vi "svx_Waterfall ZUnitsToIndex.vi"(8 "Rounding Type":T1(ring), 9 "dz":dbl, 10 "z0":dbl, 11 "Z In Units":dbl) -> (3 "ZIndex":i32)   [LabVIEW 2017, in "SVX Waterfall Graph.xctl"]
uses:
  <vilib>/addons/_XControls/Waterfall Graph/SVX Waterfall Graph.xctl
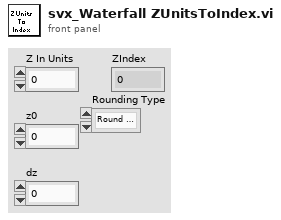
[diagram p1: front panel]
types:
  T1 = enum16{"Round To Nearest", "Round To -Inf", "Round to + Inf"}
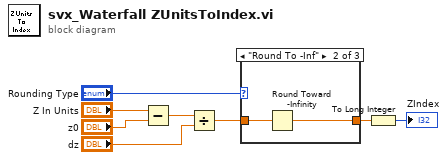
[diagram p0: block diagram]
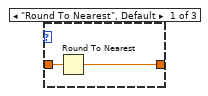
[diagram p2: hidden frame]
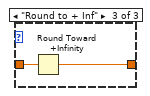
[diagram p3: hidden frame]
diagram:
  n1 = Subtract(x="Z In Units", y="z0") -> (x-y=w5:dbl)
  n2 = Divide(x=w5, y="dz") -> (x/y=w3:dbl)
  n3 = case shown="\"Round To -Inf\"" "Rounding Type" {
    tunnel: w3 -> [w10 w12 w14]
    tunnel: [w9 w11 w13] -> w1
    frame "Round To Nearest", Default {
      n4 = Round To Nearest(number=w10) -> (nearest integer value=w9:dbl)
    }
    frame "Round To -Inf" {
      n5 = Round Toward -Infinity(1:w12) -> (0:w11:dbl)
    }
    frame "Round to + Inf" {
      n6 = Round Toward +Infinity(x=w14) -> (ceil(x): smallest int >= x=w13:dbl)
    }
  }
  n7 = To Long Integer(number=w1) -> (32bit integer=→"ZIndex":i32)
